vi "10 Kwh battery decode Sub.vi"(10 "Batter Data":string) -> (2 "Data out":dbl[](array[numeric]))   [LabVIEW 2021]
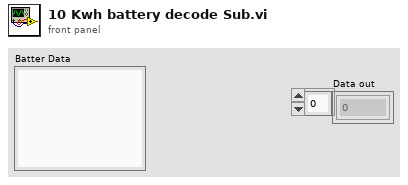
[diagram p1: front panel]
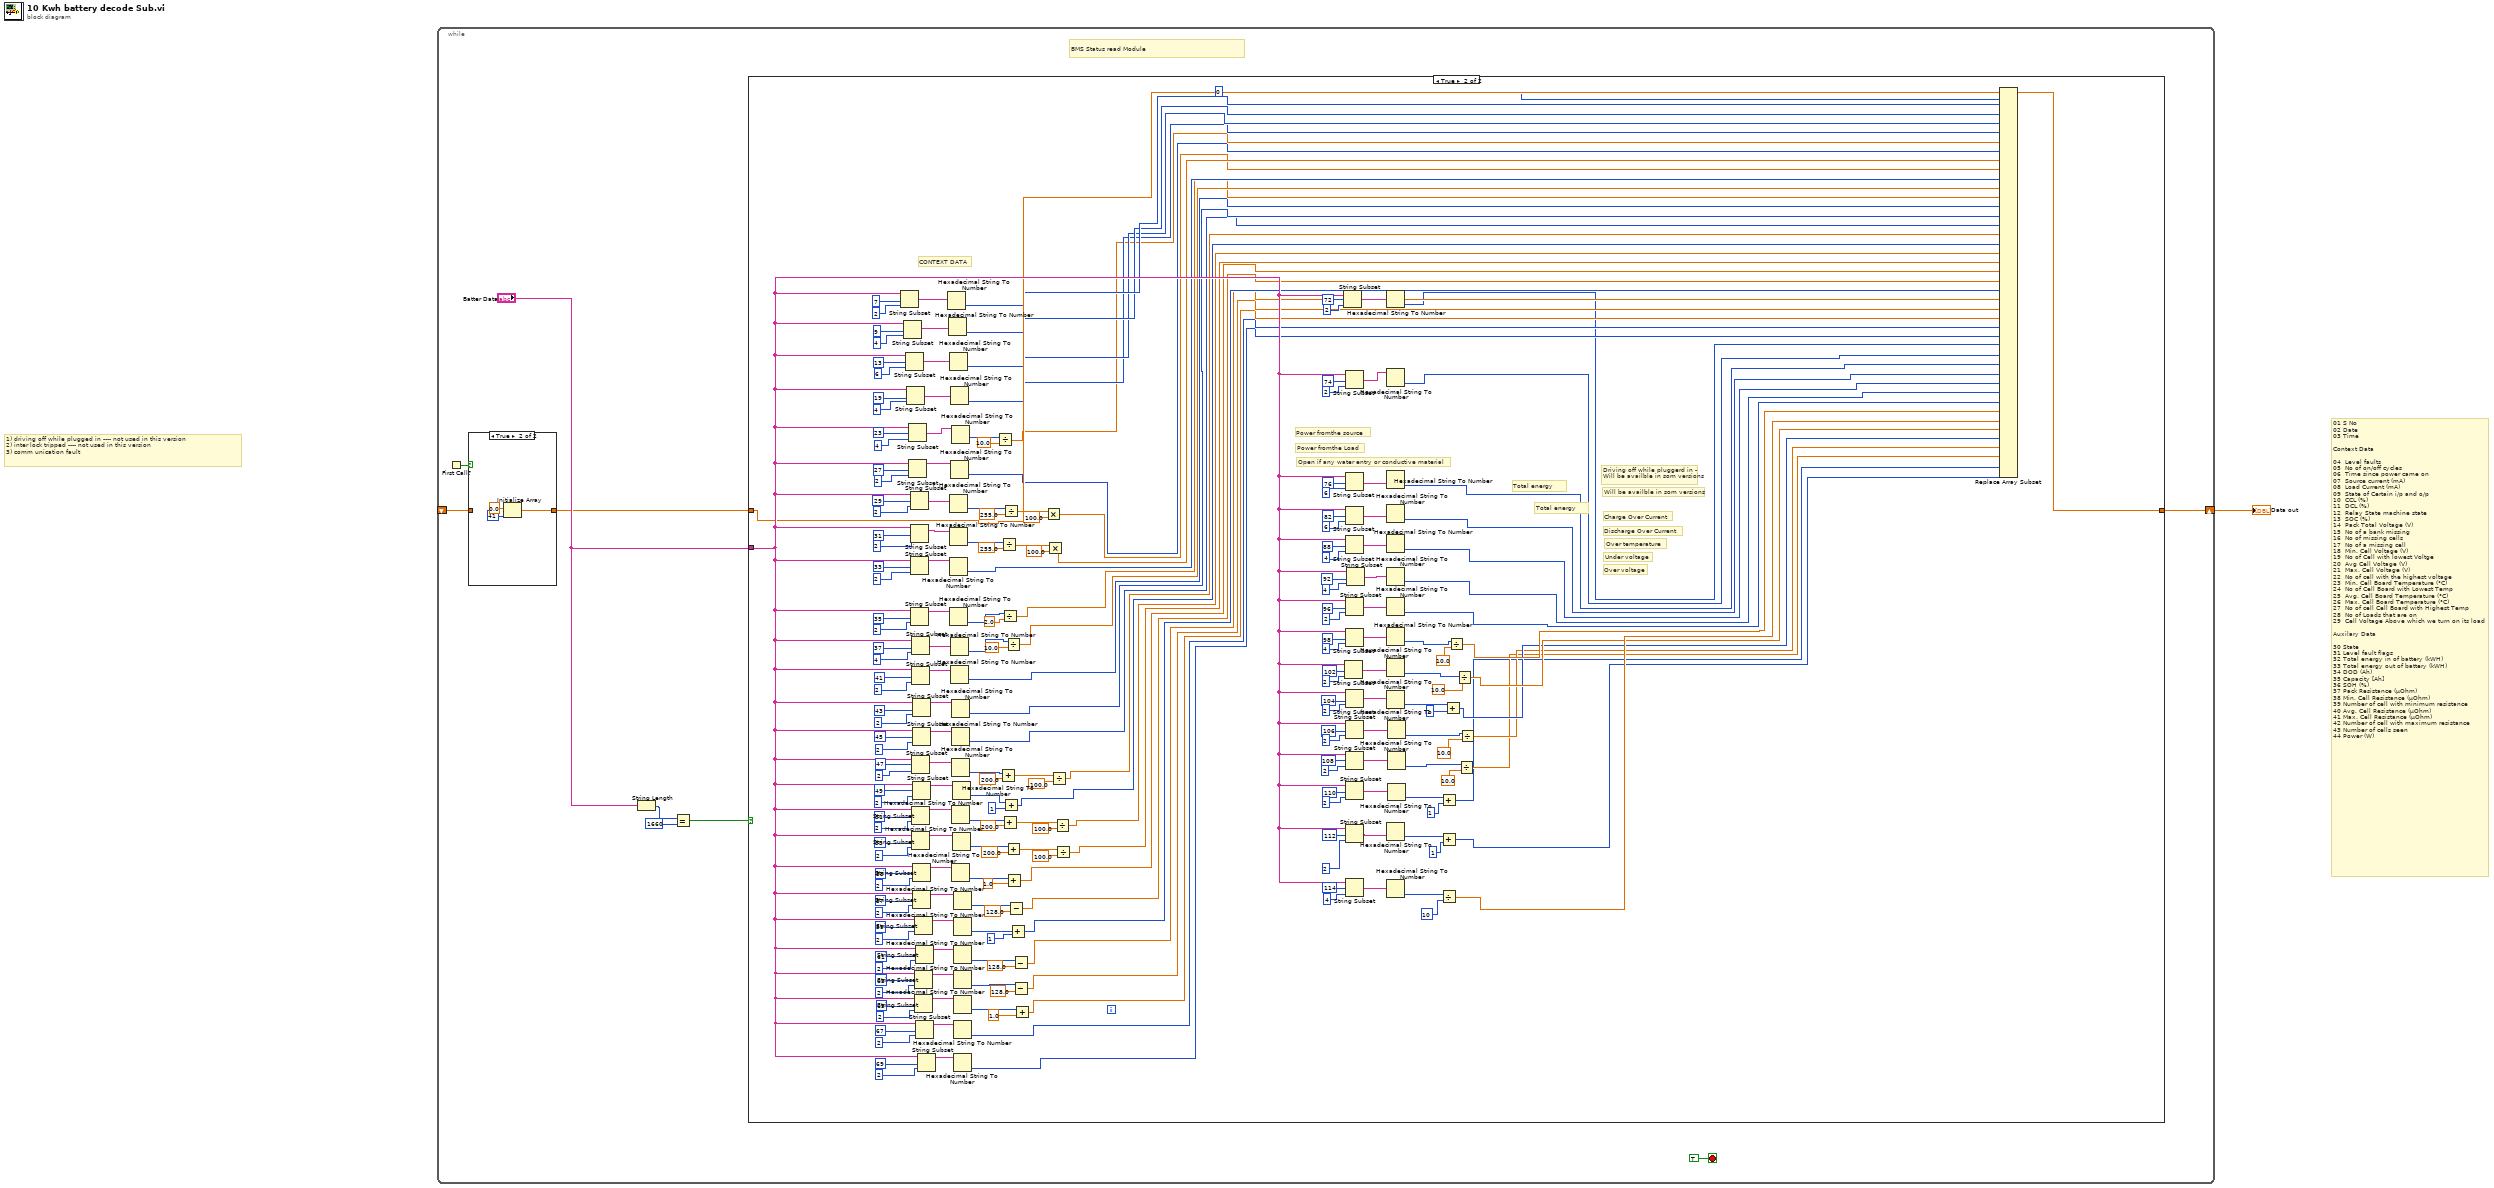
[diagram p0: block diagram]
diagram:
  # "1) driving off while plugged in ---- not used in this version\n2) inter lock tripped ---- not used in this version\n3) comm unication fault"
  # "01 S No\n02 Date\n03 Time\n\nContext Data\n\n04  Level faults\n05  No of on/off cycles\n06  Time since power came on\n07  Source current (mA)\n08  Load Current (mA)\n09  State of Certain i/p and o/p\n10  CCL (%)\n11  DCL (%)\n12  Relay State machine state\n13  SOC (%)\n14  Pack Total Voltage (V)\n15  No of a bank missing\n16  No of missing cells\n17  No of a missing cell\n18  Min. Cell Voltage (V)\n19  No of Cell with lowest Voltge\n20  Avg Cell Voltage (V)\n21  Max. Cell Voltage (V)\n22  No of cell with the highest voltage\n23  Min. Cell Board Temperature (°C)\n24  No of Cell Board with Lowest Temp\n25  Avg. Cell Board Temperature (°C)\n26  Max. Cell Board Temperature (°C)\n27  No of cell Cell Board with Highest Temp\n28  No of Loads that are on\n29  Cell Voltage Above which we turn on its load \n\nAuxilary Data\n\n30 State\n31 Level fault flags\n32 Total energy in of battery (kWH)\n33 Total energy out of battery (kWH)\n34 DOD (Ah)\n35 Capacity [Ah] \n36 SOH (%)\n37 Pack Resistance (µOhm)\n38 Min. Cell Resistance (µOhm)\n39 Number of cell with minimum resistance\n40 Avg. Cell Resistance (µOhm)  \n41 Max. Cell Resistance (µOhm) \n42 Number of cell with maximum resistance\n43 Number of cells seen\n44 Power (W)"
  n1 = while {
    shift-right: [w2] -> w1
    shift-left: _ -> [w4]
    stop <- TRUE stop-if-true
    # "BMS Status read Module"
    n2 = First Call?() -> (First Call?: T/F=w5:bool)
    n3 = case shown="True" w5 {
      tunnel: [w11 w12] -> w3
      tunnel: w4 -> [w11 _]
      frame False {
      }
      frame True {
        n4 = Initialize Array(0.0 ("element"), 41 ("dimension size")) -> (w12:dbl[])
      }
    }
    n5 = String Length(string="Batter Data") -> (length=w10:i32)
    n6 = Equal?(x=w10, y=1660) -> (x = y?=w8:bool)
    n7 = case shown="True" w8 {
      tunnel: "Batter Data" -> [_ w66]
      tunnel: w3 -> [w15 w59]
      tunnel: [w15 w58] -> w2
      frame False {
      }
      frame True {
        # "Will be availble in som versions"
        # "Open if any water entry or conductive material"
        # "Power fromthe Load"
        # "Power fromthe source"
        # "Driving off while pluggerd in -  Will be availble in som versions"
        # "Discharge Over Current"
        # "Over voltage"
        # "Under voltage"
        # "Charge Over Current"
        # "Over temperature"
        # "Total energy"
        # "Total energy"
        # "CONTEXT DATA"
        n8 = String Subset(string=w66, offset (0)=7, length (rest)=2 ("length (rest)")) -> (substring=w237:string)
        n9 = String Subset(string=w66, offset (0)=9, length (rest)=4 ("length (rest)")) -> (substring=w235:string)
        n10 = String Subset(string=w66, offset (0)=13, length (rest)=6 ("length (rest)")) -> (substring=w232:string)
        n11 = String Subset(string=w66, offset (0)=19, length (rest)=4 ("length (rest)")) -> (substring=w185:string)
        n12 = String Subset(string=w66, offset (0)=23, length (rest)=4 ("length (rest)")) -> (substring=w183:string)
        n13 = String Subset(string=w66, offset (0)=27, length (rest)=2 ("length (rest)")) -> (substring=w184:string)
        n14 = String Subset(string=w66, offset (0)=31, length (rest)=2 ("length (rest)")) -> (substring=w181:string)
        n15 = String Subset(string=w66, offset (0)=33, length (rest)=2 ("length (rest)")) -> (substring=w180:string)
        n16 = String Subset(string=w66, offset (0)=35, length (rest)=2 ("length (rest)")) -> (substring=w179:string)
        n17 = String Subset(string=w66, offset (0)=29, length (rest)=2 ("length (rest)")) -> (substring=w182:string)
        n18 = String Subset(string=w66, offset (0)=37, length (rest)=4 ("length (rest)")) -> (substring=w178:string)
        n19 = String Subset(string=w66, offset (0)=41, length (rest)=2 ("length (rest)")) -> (substring=w177:string)
        n20 = String Subset(string=w66, offset (0)=47, length (rest)=2 ("length (rest)")) -> (substring=w174:string)
        n21 = String Subset(string=w66, offset (0)=51, length (rest)=2 ("length (rest)")) -> (substring=w172:string)
        n22 = String Subset(string=w66, offset (0)=53, length (rest)=2 ("length (rest)")) -> (substring=w171:string)
        n23 = String Subset(string=w66, offset (0)=45, length (rest)=2 ("length (rest)")) -> (substring=w175:string)
        n24 = String Subset(string=w66, offset (0)=49, length (rest)=2 ("length (rest)")) -> (substring=w173:string)
        n25 = String Subset(string=w66, offset (0)=43, length (rest)=2 ("length (rest)")) -> (substring=w176:string)
        n26 = String Subset(string=w66, offset (0)=55, length (rest)=2 ("length (rest)")) -> (substring=w169:string)
        n27 = String Subset(string=w66, offset (0)=57, length (rest)=2 ("length (rest)")) -> (substring=w168:string)
        n28 = String Subset(string=w66, offset (0)=59, length (rest)=2 ("length (rest)")) -> (substring=w167:string)
        n29 = String Subset(string=w66, offset (0)=63, length (rest)=2 ("length (rest)")) -> (substring=w165:string)
        n30 = String Subset(string=w66, offset (0)=65, length (rest)=2 ("length (rest)")) -> (substring=w164:string)
        n31 = String Subset(string=w66, offset (0)=61, length (rest)=2 ("length (rest)")) -> (substring=w166:string)
        n32 = String Subset(string=w66, offset (0)=67, length (rest)=2 ("length (rest)")) -> (substring=w163:string)
        n33 = String Subset(string=w66, offset (0)=69, length (rest)=2 ("length (rest)")) -> (substring=w162:string)
        n34 = Hexadecimal String To Number(string=w237) -> (number=w56:u32)  [unwired: 2 in, 1 out]
        n35 = Hexadecimal String To Number(string=w235) -> (number=w55:u32)  [unwired: 2 in, 1 out]
        n36 = Hexadecimal String To Number(string=w232) -> (number=w54:u32)  [unwired: 2 in, 1 out]
        n37 = Hexadecimal String To Number(string=w182) -> (number=w158:u32)  [unwired: 2 in, 1 out]
        n38 = Hexadecimal String To Number(string=w181) -> (number=w152:u32)  [unwired: 2 in, 1 out]
        n39 = Hexadecimal String To Number(string=w180) -> (number=w48:u32)  [unwired: 2 in, 1 out]
        n40 = Hexadecimal String To Number(string=w179) -> (number=w150:u32)  [unwired: 2 in, 1 out]
        n41 = Hexadecimal String To Number(string=w178) -> (number=w148:u32)  [unwired: 2 in, 1 out]
        n42 = Hexadecimal String To Number(string=w177) -> (number=w45:u32)  [unwired: 2 in, 1 out]
        n43 = Hexadecimal String To Number(string=w185) -> (number=w53:u32)  [unwired: 2 in, 1 out]
        n44 = Hexadecimal String To Number(string=w184) -> (number=w51:u32)  [unwired: 2 in, 1 out]
        n45 = Hexadecimal String To Number(string=w183) -> (number=w160:u32)  [unwired: 2 in, 1 out]
        n46 = Hexadecimal String To Number(string=w172) -> (number=w142:u32)  [unwired: 2 in, 1 out]
        n47 = Hexadecimal String To Number(string=w176) -> (number=w44:u32)  [unwired: 2 in, 1 out]
        n48 = Hexadecimal String To Number(string=w175) -> (number=w43:u32)  [unwired: 2 in, 1 out]
        n49 = Hexadecimal String To Number(string=w174) -> (number=w146:u32)  [unwired: 2 in, 1 out]
        n50 = Hexadecimal String To Number(string=w169) -> (number=w130:u32)  [unwired: 2 in, 1 out]
        n51 = Hexadecimal String To Number(string=w173) -> (number=w70:u32)  [unwired: 2 in, 1 out]
        n52 = Hexadecimal String To Number(string=w171) -> (number=w138:u32)  [unwired: 2 in, 1 out]
        n53 = Hexadecimal String To Number(string=w168) -> (number=w128:u32)  [unwired: 2 in, 1 out]
        n54 = Hexadecimal String To Number(string=w167) -> (number=w133:u32)  [unwired: 2 in, 1 out]
        n55 = Hexadecimal String To Number(string=w166) -> (number=w126:u32)  [unwired: 2 in, 1 out]
        n56 = Hexadecimal String To Number(string=w165) -> (number=w124:u32)  [unwired: 2 in, 1 out]
        n57 = Hexadecimal String To Number(string=w164) -> (number=w134:u32)  [unwired: 2 in, 1 out]
        n58 = Hexadecimal String To Number(string=w163) -> (number=w32:u32)  [unwired: 2 in, 1 out]
        n59 = Hexadecimal String To Number(string=w162) -> (number=w31:u32)  [unwired: 2 in, 1 out]
        n60 = Divide(x=w160, y=10.0) -> (x/y=w52:dbl)
        n61 = Add(x=w146, y=200.0) -> (x+y=w145:dbl)
        n62 = Divide(x=w152, y=255.0) -> (x/y=w155:dbl)
        n63 = Divide(x=w150, y=2.0) -> (x/y=w47:dbl)
        n64 = Add(x=w142, y=200.0) -> (x+y=w141:dbl)
        n65 = Divide(x=w158, y=255.0) -> (x/y=w157:dbl)
        n66 = Add(x=w70, y=u32 1) -> (x+y=w41:u32)
        n67 = Divide(x=w148, y=10.0) -> (x/y=w46:dbl)
        n68 = Add(x=w138, y=200.0) -> (x+y=w136:dbl)
        n69 = Add(x=w130, y=1.0) -> (x+y=w38:dbl)
        n70 = Subtract(x=w128, y=128.0) -> (x-y=w37:dbl)
        n71 = Add(x=w133, y=u32 1) -> (x+y=w36:u32)
        n72 = Subtract(x=w126, y=128.0) -> (x-y=w35:dbl)
        n73 = Subtract(x=w124, y=128.0) -> (x-y=w34:dbl)
        n74 = Add(x=w134, y=1.0) -> (x+y=w33:dbl)
        n75 = Multiply(x=w157, y=100.0) -> (x*y=w50:dbl)
        n76 = Multiply(x=w155, y=100.0) -> (x*y=w49:dbl)
        n77 = Divide(x=w145, y=100.0) -> (x/y=w42:dbl)
        n78 = Divide(x=w141, y=100.0) -> (x/y=w40:dbl)
        n79 = Divide(x=w136, y=100.0) -> (x/y=w39:dbl)
        n80 = String Subset(string=w66, offset (0)=72, length (rest)=2 ("length (rest)")) -> (substring=w122:string)
        n81 = String Subset(string=w66, offset (0)=102, length (rest)=2 ("length (rest)")) -> (substring=w98:string)
        n82 = String Subset(string=w66, offset (0)=74, length (rest)=2 ("length (rest)")) -> (substring=w119:string)
        n83 = String Subset(string=w66, offset (0)=76, length (rest)=6 ("length (rest)")) -> (substring=w116:string)
        n84 = String Subset(string=w66, offset (0)=82, length (rest)=6 ("length (rest)")) -> (substring=w113:string)
        n85 = String Subset(string=w66, offset (0)=88, length (rest)=4 ("length (rest)")) -> (substring=w110:string)
        n86 = String Subset(string=w66, offset (0)=96, length (rest)=2 ("length (rest)")) -> (substring=w104:string)
        n87 = String Subset(string=w66, offset (0)=98, length (rest)=4 ("length (rest)")) -> (substring=w101:string)
        n88 = String Subset(string=w66, offset (0)=104, length (rest)=2 ("length (rest)")) -> (substring=w95:string)
        n89 = String Subset(string=w66, offset (0)=112, length (rest)=2 ("length (rest)")) -> (substring=w83:string)
        n90 = String Subset(string=w66, offset (0)=106, length (rest)=2 ("length (rest)")) -> (substring=w92:string)
        n91 = String Subset(string=w66, offset (0)=108, length (rest)=2 ("length (rest)")) -> (substring=w89:string)
        n92 = String Subset(string=w66, offset (0)=110, length (rest)=2 ("length (rest)")) -> (substring=w86:string)
        n93 = String Subset(string=w66, offset (0)=114, length (rest)=4 ("length (rest)")) -> (substring=w80:string)
        n94 = String Subset(string=w66, offset (0)=92, length (rest)=4 ("length (rest)")) -> (substring=w107:string)
        n95 = Hexadecimal String To Number(string=w122) -> (number=w30:u32)  [unwired: 2 in, 1 out]
        n96 = Hexadecimal String To Number(string=w119) -> (number=w29:u32)  [unwired: 2 in, 1 out]
        n97 = Hexadecimal String To Number(string=w116) -> (number=w28:u32)  [unwired: 2 in, 1 out]
        n98 = Hexadecimal String To Number(string=w113) -> (number=w27:u32)  [unwired: 2 in, 1 out]
        n99 = Hexadecimal String To Number(string=w110) -> (number=w26:u32)  [unwired: 2 in, 1 out]
        n100 = Hexadecimal String To Number(string=w107) -> (number=w25:u32)  [unwired: 2 in, 1 out]
        n101 = Hexadecimal String To Number(string=w104) -> (number=w24:u32)  [unwired: 2 in, 1 out]
        n102 = Hexadecimal String To Number(string=w101) -> (number=w63:u32)  [unwired: 2 in, 1 out]
        n103 = Hexadecimal String To Number(string=w98) -> (number=w62:u32)  [unwired: 2 in, 1 out]
        n104 = Hexadecimal String To Number(string=w95) -> (number=w67:u32)  [unwired: 2 in, 1 out]
        n105 = Hexadecimal String To Number(string=w83) -> (number=w79:u32)  [unwired: 2 in, 1 out]
        n106 = Hexadecimal String To Number(string=w80) -> (number=w72:u32)  [unwired: 2 in, 1 out]
        n107 = Hexadecimal String To Number(string=w92) -> (number=w61:u32)  [unwired: 2 in, 1 out]
        n108 = Hexadecimal String To Number(string=w89) -> (number=w60:u32)  [unwired: 2 in, 1 out]
        n109 = Hexadecimal String To Number(string=w86) -> (number=w77:u32)  [unwired: 2 in, 1 out]
        n110 = Add(x=w77, y=u32 1) -> (x+y=w17:u32)
        n111 = Add(x=w79, y=u32 1) -> (x+y=w16:u32)
        n112 = Divide(x=w72, y=u32 10) -> (x/y=w22:dbl)
        n113 = Add(x=w67, y=u32 1) -> (x+y=w20:u32)
        n114 = Divide(x=w63, y=10.0) -> (x/y=w23:dbl)
        n115 = Divide(x=w62, y=10.0) -> (x/y=w21:dbl)
        n116 = Divide(x=w60, y=10.0) -> (x/y=w18:dbl)
        n117 = Divide(x=w61, y=10.0) -> (x/y=w19:dbl)
        n118 = Replace Array Subset(array=w59, new element #1=w56, index #1=0 ("index"), new element #2=w55, new element #3=w54, new element #4=w53, new element #5=w52, new element #6=w51, new element #7=w50, new element #8=w49, new element #9=w48, new element #10=w47, new element #11=w46, new element #12=w45, new element #13=w44, new element #14=w43, new element #15=w42, new element #16=w41, new element #17=w40, new element #18=w39, new element #19=w38, new element #20=w37, new element #21=w36, new element #22=w35, new element #23=w34, new element #24=w33, new element #25=w32, new element #26=w31, new element #27=w30, new element #28=w29, new element #29=w28, new element #30=w27, new element #31=w26, new element #32=w25, new element #33=w24, new element #34=w23, new element #35=w22, new element #36=w21, new element #37=w20, new element #38=w19, new element #39=w18, new element #40=w17, new element #41=w16) -> (w58:dbl[])  [unwired: 40 in]
      }
    }
  }
  "Data out" <- w1
